vi "Get Filtered XNET Change List.vi"(10 "VS Existing Frames":T1[](array[typedef]) {"Node Ref" format="%.0x"}, 11 "XNET Change List":T9) -> (3 "Filtered VS Change List":T4 {"Missing"."Node Ref" format="%.0x"; "Changed"."Old"."Node Ref" format="%.0x"})   [LabVIEW 2025, in "Protection and Counter Addon System Explorer.lvlib"]
uses:
  Protection and Counter Addon System Explorer.lvlib
  Types/XNET Change List.ctl
  Types/Base Frame Info_NoVS.ctl
  Types/Signal Attributes.ctl
  Types/CAN Filter Type.ctl
  Types/Related CAN Frames No VS.ctl
  Types/Database Changes.ctl
  Types/Base Frame Info.ctl
  <vilib>/NI VeriStand/Custom Device API/Custom Device Item Ref.ctl
  Types/Related CAN Frames.ctl
  <vilib>/NI VeriStand/Custom Device API/Custom Device API.lvlib
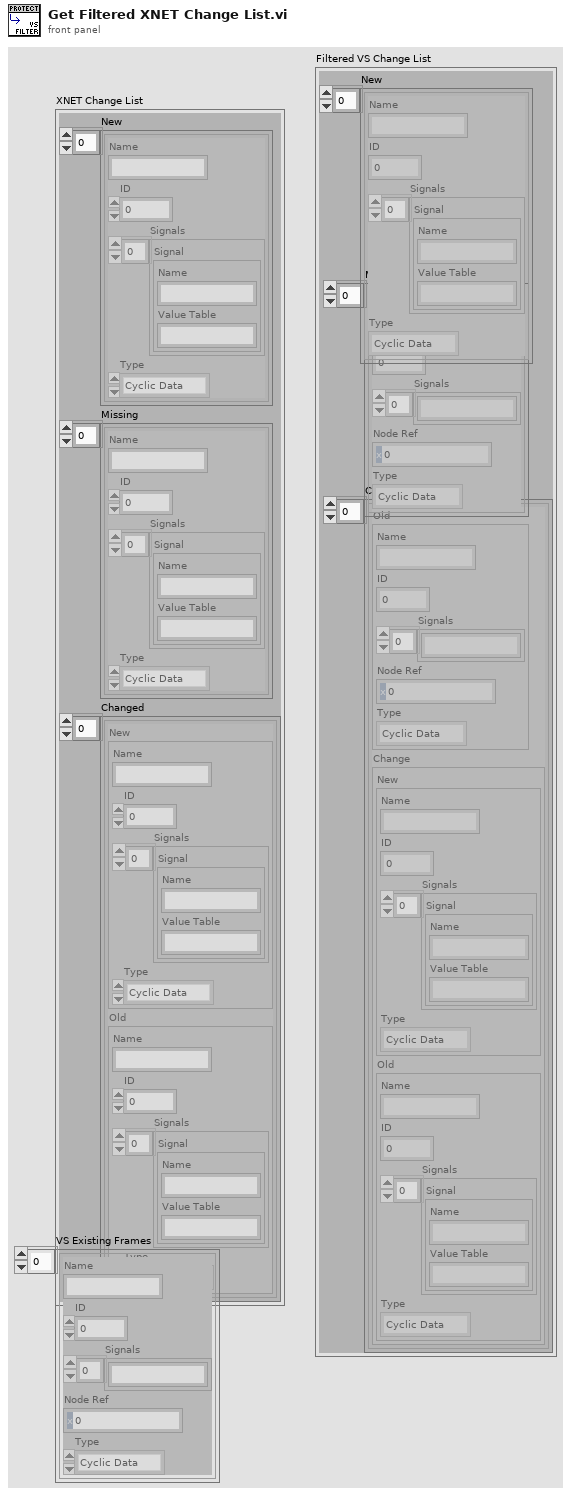
[diagram p1: front panel]
types:
  T1 = typedef "Protection and Counter Addon System Explorer.lvlib/Base Frame Info.ctl" = cluster{"Name":string, "ID":u32, "Signals":string[], "Node Ref":T2, "Type":T3}
  T2 = typedef "Custom Device API.lvlib/Custom Device Item Ref.ctl" = u64
  T3 = typedef "Protection and Counter Addon System Explorer.lvlib/CAN Filter Type.ctl" = enum16{"Cyclic Data", "Event Data", "Cyclic/Event", "All"}
  T4 = typedef "Protection and Counter Addon System Explorer.lvlib/Database Changes.ctl" = cluster{"New":T5[], "Missing":T1[], "Changed":T7[]}
  T5 = typedef "Protection and Counter Addon System Explorer.lvlib/Base Frame Info_NoVS.ctl" = cluster{"Name":string, "ID":u32, "Signals":T6[], "Type":T3}
  T6 = typedef "Protection and Counter Addon System Explorer.lvlib/Signal Attributes.ctl" = cluster{"Name":string, "Value Table":string}
  T7 = typedef "Protection and Counter Addon System Explorer.lvlib/Related CAN Frames.ctl" = cluster{"Old":T1, "Change":T8}
  T8 = typedef "Protection and Counter Addon System Explorer.lvlib/Related CAN Frames No VS.ctl" = cluster{"New":T5, "Old":T5}
  T9 = typedef "Protection and Counter Addon System Explorer.lvlib/XNET Change List.ctl" = cluster{"New":T5[], "Missing":T5[], "Changed":T8[]}
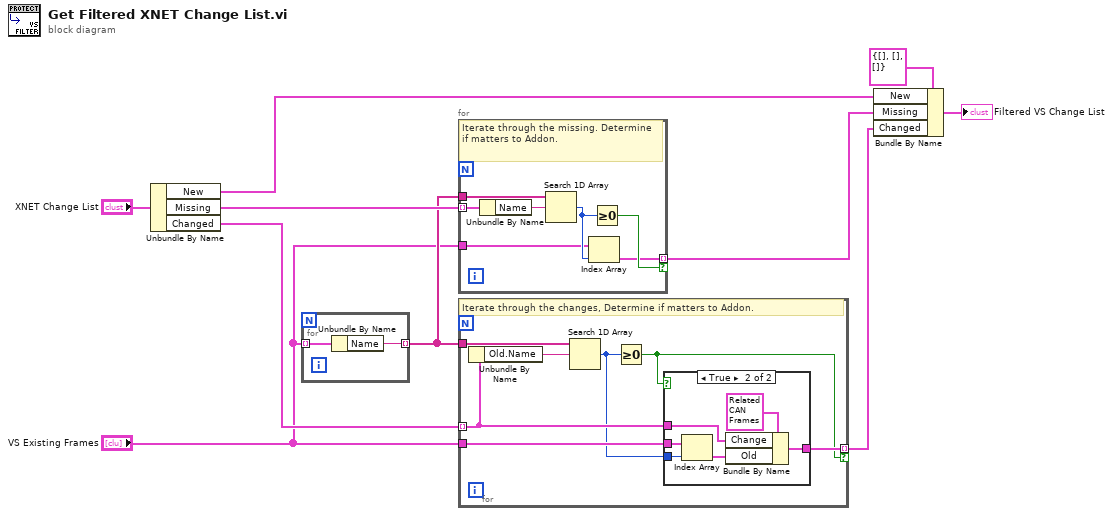
[diagram p0: block diagram]
diagram:
  n1 = Unbundle By Name("XNET Change List") -> ("New"=w8:T5[], "Missing"=w9:T5[], "Changed"=w10:T8[])
  n2 = for {
    tunnel: "VS Existing Frames" -> [w12] mode=indexing
    tunnel: [w11] -> w2 mode=indexing
    n3 = Unbundle By Name(w12) -> ("Name"=w11:string)
  }
  n4 = for {
    tunnel: w9 -> [w18] mode=indexing
    tunnel: w2 -> [w17]
    tunnel: [w13] -> w3 mode=indexing if=w16
    tunnel: "VS Existing Frames" -> [w14]
    # "Iterate through the missing. Determine if matters to Addon."
    n5 = Unbundle By Name(w18) -> ("Name"=w19:string)
    n6 = Search 1D Array(1D array=w17, element=w19) -> (index of element=w15:i32)  [unwired: 1 in]
    n7 = Index Array(array=w14, index=w15) -> (element=w13:T1)
    n8 = Greater Or Equal To 0?(x=w15) -> (x >= 0?=w16:bool)
  }
  n9 = for {
    tunnel: w10 -> [w22] mode=indexing
    tunnel: w2 -> [w25]
    tunnel: "VS Existing Frames" -> [w24]
    tunnel: [w23] -> w4 mode=indexing if=w21
    # "Iterate through the changes, Determine if matters to Addon."
    n10 = Unbundle By Name(w22) -> ("Old.Name"=w26:string)
    n11 = Search 1D Array(1D array=w25, element=w26) -> (index of element=w20:i32)  [unwired: 1 in]
    n12 = Greater Or Equal To 0?(x=w20) -> (x >= 0?=w21:bool)
    n13 = case shown="True" w21 {
      tunnel: w24 -> [_ w32]
      tunnel: w20 -> [_ w31]
      tunnel: [_ w30] -> w23
      tunnel: w22 -> [_ w29]
      frame False {
      }
      frame True {
        n14 = Index Array(array=w32, index=w31) -> (element=w27:T1)
        n15 = Bundle By Name(cluster=T7 {"Old"={"Name"="", "ID"=0, "Signals"=[], "Node Ref"=0, "Type"=enum."Cyclic Data"}, "Change"={"New"={"Name"="", "ID"=0, "Signals"=[], "Type"=enum."Cyclic Data"}, "Old"={"Name"="", "ID"=0, "Signals"=[], "Type"=enum."Cyclic Data"}}}, "Change"=w29, "Old"=w27) -> (w30:T7)
      }
    }
  }
  n16 = Bundle By Name(cluster=T4 {"New"=[], "Missing"=[], "Changed"=[]}, "New"=w8, "Missing"=w3, "Changed"=w4) -> (→"Filtered VS Change List":T4)
